vi "Handle Error.vi"(8 "error in (no error)":errorcluster, 11 "Sim User Console Actor in":refnum<class "Sim User Console Actor.lvclass">) -> (0 "error out":errorcluster, 2 "stop actor?":bool=TRUE, 3 "Sim User Console Actor out":refnum<class "Sim User Console Actor.lvclass">)   [LabVIEW 2022 SP3, in "Sim User Console Actor.lvlib" / "Sim User Console Actor.lvclass"]
doc: "(<B>Filename</B>: Actor Framework.lvlib:Actor.lvclass:Handle Error.vi)\n\nDefines how the actor handles an error that occurred while processing a message.\n\nBy default, this method does nothing except stop the actor. This method also treats error code 43 (coming from <B>error in</B>) as a sign that the actor shut down normally. In this situation, the Handle Error method does not return the error on <B>error out</B>, meaning the actor's caller will not receive it. All other error codes will be returned on <B>error out</B>.\n\nA descendant class may override this method to change this behavior."
uses:
  Sim User Console Actor.lvclass
  Abstract User Console Actor/Abstract User Console Actor/Abstract User Console Actor.lvclass
  Sim User Console Actor.lvclass/Sim User Console Actor.ctl
  Elevator Controller/Elevator Controller Messages/Centralize Error Msg/Centralize Error Msg.lvclass
  <vilib>/ActorFramework/Actor/Actor.lvclass
  C:/Workspace/CLA/Elevator AF_2022/Abstract User Console Actor/Abstract User Console Actor/Abstract User Console Actor.lvclass
  C:/Program Files/National Instruments/LabVIEW 2022/vi.lib/ActorFramework/Actor/Actor.lvclass
  C:/Workspace/CLA/Elevator AF_2022/Sim User Console Actor/Abstract User Console Actor/Sim User Console Actor.lvclass
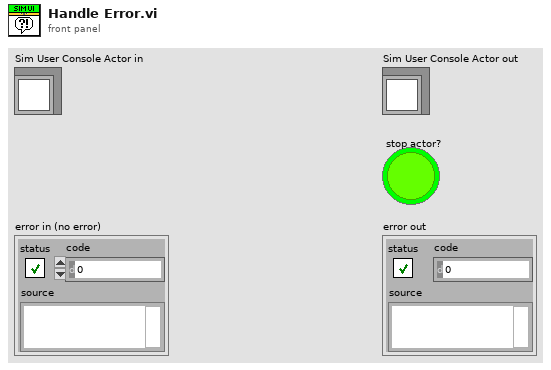
[diagram p1: front panel]
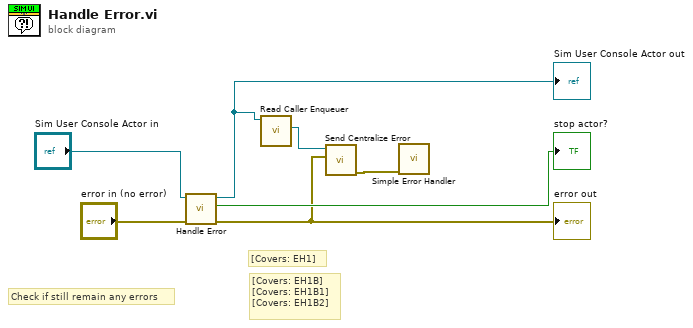
[diagram p0: block diagram]
diagram:
  # "Check if still remain any errors"
  # "[Covers: EH1B] \n[Covers: EH1B1] \n[Covers: EH1B2]"
  # "[Covers: EH1]"
  n1 = call-parent "Handle Error.vi"("error in (no error)"="error in (no error)", "Actor in"="Sim User Console Actor in") -> ("error out"=w4:errorcluster, "stop actor?"=→"stop actor?":bool, "Actor out"=w3:refnum<class "Sim User Console Actor.lvclass">)  [unwired: 7 in]
  "Sim User Console Actor out" <- w3
  "error out" <- w4
  n2 = call <vilib>:"Read Caller Enqueuer.vi"("Actor"=w3) -> ("Caller Enqueuer"=w2:refnum<class "Message Enqueuer.lvclass">)  [unwired: 10 in]
  n3 = call "Send Centralize Error.vi"("Error"=w4, "Message Enqueuer"=w2) -> ("error out"=w1:errorcluster)  [unwired: 8 in, 1 out]
  n4 = call <vilib>:"Simple Error Handler.vi"("error in (no error)"=w1) -> ()  [unwired: 4 in, 5 out]
